vi "SFCS_GET_IMEI_IPEI_CMP_LBL.vi"() -> ()   [LabVIEW 2011]
uses:
  Instance           4 34Saved   SFCS_GET_IMEI_IPEI_CMP_LBL .vi
  Instance           8 34Saved   SFCS_GET_IMEI_IPEI_CMP_LBL .vi
  Instance           9 34Saved   SFCS_GET_IMEI_IPEI_CMP_LBL .vi
  Instance          10 34Saved   SFCS_GET_IMEI_IPEI_CMP_LBL .vi
  Instance          11 34Saved   SFCS_GET_IMEI_IPEI_CMP_LBL .vi
  Instance          14 34Saved   SFCS_GET_IMEI_IPEI_CMP_LBL .vi
panel:
  out "Found barcode label info?":bool
  out "IPEI_IMEI_Label":string
  out "SFCS_IPEI_IMEI":string
  out "SN":string
  out "SeqNo":i32
  out "Sequence":string
  out "Category":string
  out "STAGE":string
  out "SFCS_IP":string
  out "BEGIN TIME":u32
  # "KT300W/KT300M Get IPEI /IMEI from ShopFlow\n需網路連線至ShopFlow 取得IPEI /IMEI"
  # "2013-3-28"
  # "Step1: Get the IPEI or IMEI from a remote Server by issuing SN\n\nStep2: Auto Comapre with Label content and SN of Database"
  # "系統會自動比對Shoflow 的IPEI/IMEI 是否與條碼一致"
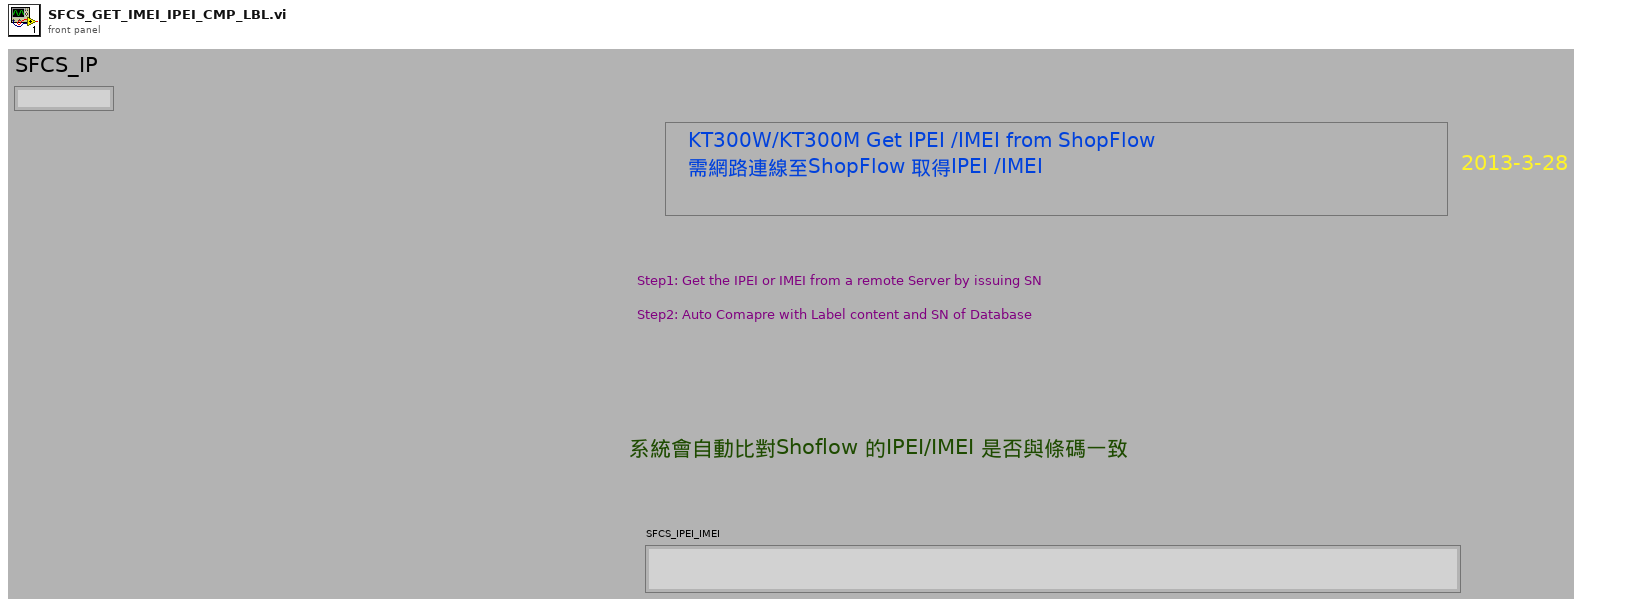
[diagram p1: front panel]
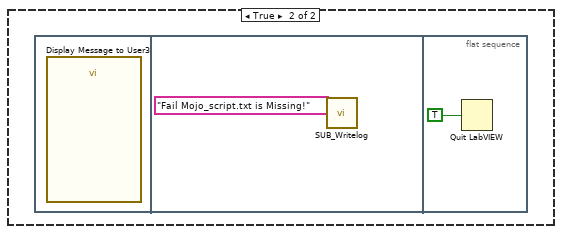
[diagram p5: hidden frame]
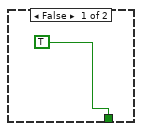
[diagram p8: hidden frame]
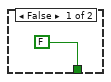
[diagram p9: hidden frame]
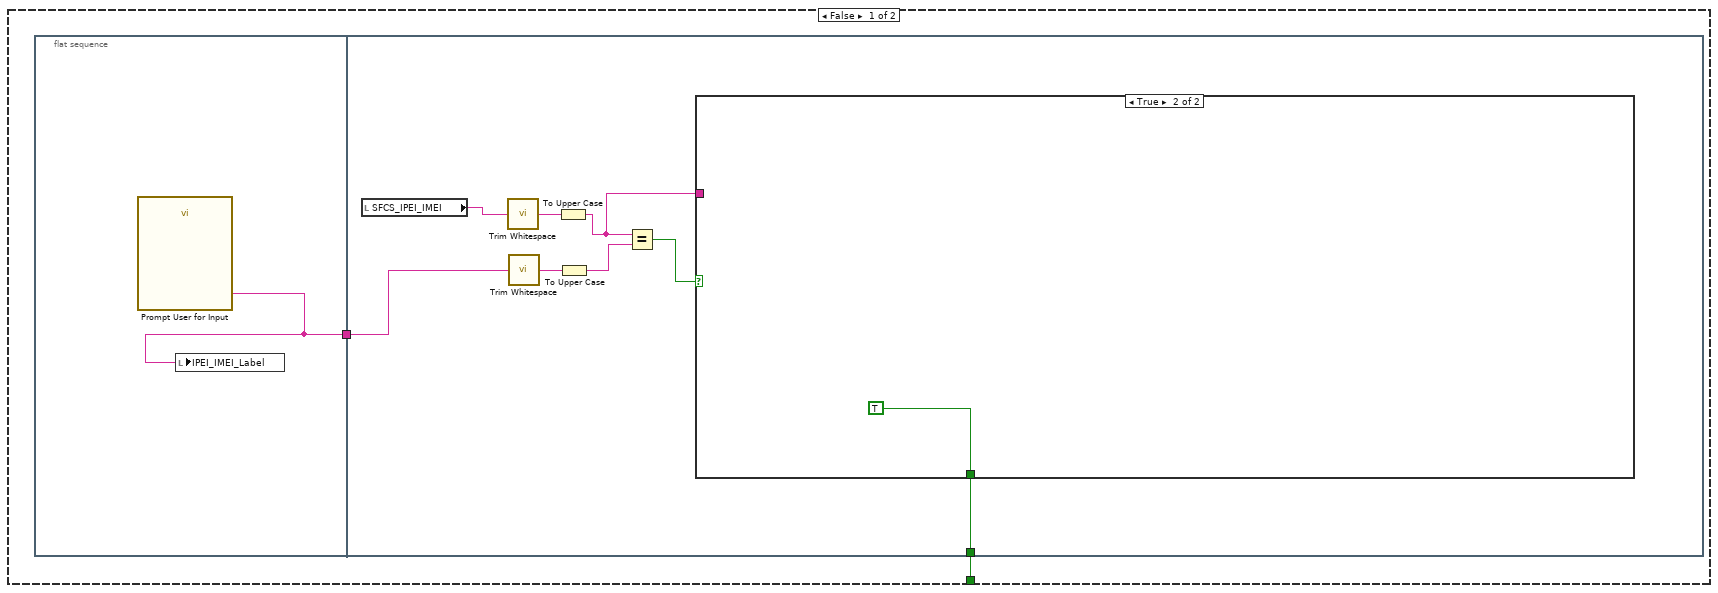
[diagram p10: hidden frame]
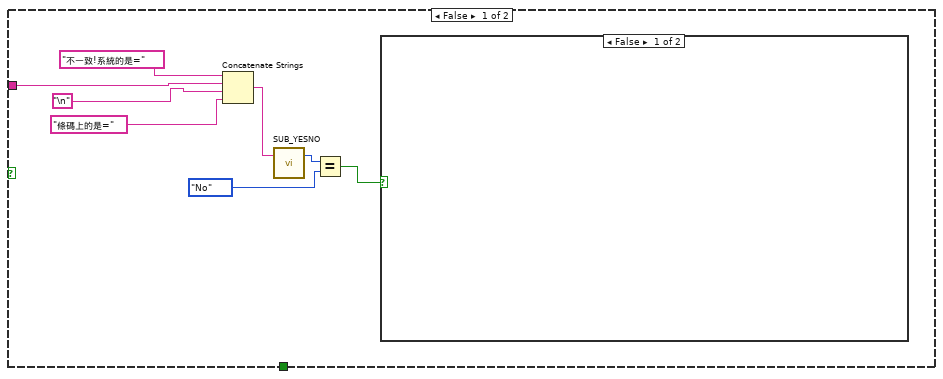
[diagram p11: hidden frame]
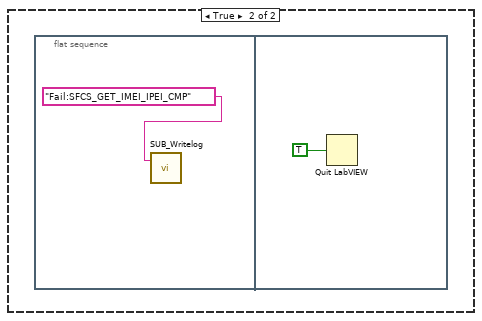
[diagram p12: hidden frame]
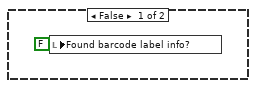
[diagram p13: hidden frame]
diagram:
  n1 = flat-sequence {
    tunnel: [w15] -> w1
    tunnel: w1 -> [w36]
    frame #0 {
      n2 = Tick Count (ms)() -> (millisecond timer value=→"BEGIN TIME":u32)
    }
    frame #1 {
      n3 = local write "Found barcode label info?"(FALSE ("Found barcode label info?")) -> ()
    }
    frame #2 {
      w4 = "barcode.LOG" ("Search Filename in Folder")
      n4 = call "SUB_SearchFile_inFolder.vi"("Search Filename in Folder"=w4) -> ("File Existing True/Flase"=w5:bool)  [unwired: 1 in]
      n5 = case shown="True" w5 {
        tunnel: w4 -> [_ w10]
        frame False {
        }
        frame True {
          n6 = call "SUB_Read_specifFile.vi"("name or relative path"=w10) -> ("text"=w9:string)  [unwired: 1 in, 1 out]
          n7 = call "SUB_FindSpecificString.vi"("Find this String"="IPEI_IMEI=", "String data"=w9) -> ("before \"; \" string"=→"IPEI_IMEI_Label":string, "Found"=→"Found barcode label info?":bool)  [unwired: 2 in]
        }
      }
    }
    frame #3 {
      n8 = call "SUB_SearchFile_inFolder.vi"("Search Filename in Folder"="SFCS_INFO.LOG") -> ("File Existing True/Flase"=w11:bool)  [unwired: 1 in]
      n9 = case shown="False" w11 {
        frame False {
          n10 = flat-sequence {
            frame #0 {
              n11 = call "Display Message to User"() -> ()  [unwired: 10 in, 2 out]
            }
            frame #1 {
              n12 = call "SUB_Writelog.vi"("Pass/Fail"="Fail :Please Do Check Route First !") -> ()  [unwired: 2 in]
            }
            frame #2 {
              n13 = Quit LabVIEW(quit? (T)=TRUE) -> ()
            }
          }
        }
        frame True {
        }
      }
    }
    frame #4 {
      n14 = call "SUB_ReadScript_File.vi"("Script FileName"="konftel_sfcs_misc.TXT") -> ("error out"=w19:errorcluster, "text"=w15:string)  [unwired: 1 in]
      n15 = Unbundle By Name(w19) -> ("code"=w18:i32)
      n16 = Not Equal To 0?(x=w18) -> (x != 0?=w17:bool)
      n17 = case shown="False" w17 {
        tunnel: w15 -> [w20 _]
        frame False {
          n18 = flat-sequence {
            tunnel: w20 -> [w26]
            frame #0 {
              n19 = To Upper Case(1:"SFCS_IP=" ("string")) -> (0:w30:string)
              n20 = To Upper Case(1:w26) -> (0:w31:string)
              n21 = call <vilib>:"Trim Whitespace.vi"("string"=w30) -> ("trimmed string"=w28:string)  [unwired: 1 in]
              n22 = call <vilib>:"Trim Whitespace.vi"("string"=w31) -> ("trimmed string"=w27:string)  [unwired: 1 in]
              n23 = Match Pattern(string=w27, regular expression=w28) -> (after substring=w25:string)  [unwired: 1 in, 3 out]
              n24 = Match Pattern(string=w25, regular expression=";") -> (before substring=w23:string)  [unwired: 1 in, 3 out]
              "SFCS_IP" <- w23
              n25 = Equal?(x=w23, y="") -> (x = y?=w21:bool)
              n26 = case shown="True" w21 {
                frame False {
                }
                frame True {
                  n27 = flat-sequence {
                    frame #0 {
                      n28 = call "Display Message to User2"() -> ()  [unwired: 10 in, 2 out]
                    }
                    frame #1 {
                      n29 = call "SUB_Writelog.vi"("Pass/Fail"="Fail Not Found SFCS_IP=\"xx.xx.xx.xx\" in Mojo_script.txt !") -> ()  [unwired: 2 in]
                    }
                    frame #2 {
                      n30 = Quit LabVIEW(quit? (T)=TRUE) -> ()
                    }
                  }
                }
              }
            }
          }
        }
        frame True {
          n31 = flat-sequence {
            frame #0 {
              n32 = call "Display Message to User3"() -> ()  [unwired: 10 in, 2 out]
            }
            frame #1 {
              n33 = call "SUB_Writelog.vi"("Pass/Fail"="Fail Mojo_script.txt is Missing!") -> ()  [unwired: 2 in]
            }
            frame #2 {
              n34 = Quit LabVIEW(quit? (T)=TRUE) -> ()
            }
          }
        }
      }
    }
    frame #5 {
      n35 = To Upper Case(1:"SFCS_STAGE=" ("string")) -> (0:w68:string)
      n36 = To Upper Case(1:w36) -> (0:w69:string)
      n37 = To Upper Case(1:"SFCS_IMEI_IPEI_Category=" ("string")) -> (0:w61:string)
      n38 = To Upper Case(1:w36) -> (0:w62:string)
      n39 = call <vilib>:"Trim Whitespace.vi"("string"=w68) -> ("trimmed string"=w67:string)  [unwired: 1 in]
      n40 = call <vilib>:"Trim Whitespace.vi"("string"=w69) -> ("trimmed string"=w66:string)  [unwired: 1 in]
      n41 = To Upper Case(1:"SFCS_Sequence=" ("string")) -> (0:w54:string)
      n42 = call <vilib>:"Trim Whitespace.vi"("string"=w61) -> ("trimmed string"=w60:string)  [unwired: 1 in]
      n43 = call <vilib>:"Trim Whitespace.vi"("string"=w62) -> ("trimmed string"=w59:string)  [unwired: 1 in]
      n44 = To Upper Case(1:w36) -> (0:w55:string)
      n45 = call <vilib>:"Trim Whitespace.vi"("string"=w54) -> ("trimmed string"=w53:string)  [unwired: 1 in]
      n46 = call <vilib>:"Trim Whitespace.vi"("string"=w55) -> ("trimmed string"=w52:string)  [unwired: 1 in]
      n47 = Match Pattern(string=w66, regular expression=w67) -> (after substring=w65:string)  [unwired: 1 in, 3 out]
      n48 = Match Pattern(string=w59, regular expression=w60) -> (after substring=w58:string)  [unwired: 1 in, 3 out]
      n49 = Match Pattern(string=w52, regular expression=w53) -> (after substring=w51:string)  [unwired: 1 in, 3 out]
      n50 = Match Pattern(string=w65, regular expression=";") -> (before substring=w48:string)  [unwired: 1 in, 3 out]
      "STAGE" <- w48
      n51 = Match Pattern(string=w58, regular expression=";") -> (before substring=w47:string)  [unwired: 1 in, 3 out]
      "Category" <- w47
      n52 = Match Pattern(string=w51, regular expression=";") -> (before substring=w38:string)  [unwired: 1 in, 3 out]
      "Sequence" <- w38
      n53 = Decimal String To Number(string=w38) -> (number=→"SeqNo":i32)  [unwired: 2 in, 1 out]
      n54 = Not Equal?(x=w47, y="") -> (x != y?=w42:bool)
      n55 = Not Equal?(x=w48, y="") -> (x != y?=w43:bool)
      n56 = Not Equal?(x=w38, y="") -> (x != y?=w40:bool)
      n57 = And(x=w43, y=w42) -> (x .and. y?=w41:bool)
      n58 = And(x=w41, y=w40) -> (x .and. y?=w39:bool)
      n59 = case shown="False" w39 {
        frame False {
          n60 = flat-sequence {
            frame #0 {
              n61 = call "Display Message to User4"() -> ()  [unwired: 10 in, 2 out]
            }
            frame #1 {
              n62 = call "SUB_Writelog.vi"("Pass/Fail"="Fail :Stage,Category,Sequence not define in script file!") -> ()  [unwired: 2 in]
            }
            frame #2 {
              n63 = Quit LabVIEW(quit? (T)=TRUE) -> ()
            }
          }
        }
        frame True {
        }
      }
    }
    frame #6 {
      n64 = call "SUB_Read_specifFile.vi"("name or relative path"="SFCS_INFO.LOG") -> ("error out"=w82:errorcluster, "text"=w81:string)  [unwired: 1 in]
      n65 = Unbundle By Name(w82) -> ("code"=w79:i32)
      n66 = call "SUB_FindSpecificString.vi"("Find this String"="USN=", "String data"=w81) -> ("before \"; \" string"=→"SN":string, "Found"=w77:bool)  [unwired: 2 in]
      n67 = Equal?(x=w79, y=0) -> (x = y?=w74:bool)
      n68 = Equal?(x=w77, y=TRUE) -> (x = y?=w75:bool)
      n69 = And(x=w75, y=w74) -> (x .and. y?=w72:bool)
      n70 = case shown="False" w72 {
        frame False {
          n71 = flat-sequence {
            frame #0 {
              n72 = call "Display Message to User5"() -> ()  [unwired: 10 in, 2 out]
            }
            frame #1 {
              n73 = call "SUB_Writelog.vi"("Pass/Fail"="Fail :Something is wrong in SFCS_INFO.LOG") -> ()  [unwired: 2 in]
            }
            frame #2 {
              n74 = Quit LabVIEW(quit? (T)=TRUE) -> ()
            }
          }
        }
        frame True {
        }
      }
    }
    frame #7 {
      n75 = while {
        stop <- w88 stop-if-true
        n76 = local read "Category"() -> (w91:string)
        n77 = local read "SeqNo"() -> (w90:i32)
        n78 = local read "SN"() -> (w93:string)
        n79 = local read "STAGE"() -> (w92:string)
        n80 = local read "SFCS_IP"() -> (w94:string)
        n81 = call "SUB_SFCS_GetUSNItem.vi"("URL"=w94, "SN"=w93, "Stage"=w92, "CATEGORY"=w91, "SEQ"=w90) -> ("Status"=w86:string)
        n82 = String Length(string=w86) -> (length=w102:i32)
        n83 = call "SUB_FindSpecificString.vi"("Find this String"="FAIL") -> ("Found"=w97:bool)  [unwired: 3 in, 1 out]
        n84 = call "SUB_FindSpecificString.vi"("Find this String"="NG", "String data"=w86) -> ("Found"=w99:bool)  [unwired: 2 in, 1 out]
        n85 = call <vilib>:"Trim Whitespace.vi"("string"=w86) -> ("trimmed string"=w96:string)  [unwired: 1 in]
        n86 = Less?(x=w102, y=3) -> (x < y?=w98:bool)
        n87 = To Upper Case(1:w96) -> (0:→"SFCS_IPEI_IMEI":string)
        n88 = Or(x=w99, y=w98) -> (x .or. y?=w89:bool)
        n89 = Or(x=w89, y=w97) -> (x .or. y?=w87:bool)
        n90 = case shown="True" w87 {
          tunnel: [TRUE w106] -> w88
          tunnel: w86 -> [_ w105]
          frame False {
          }
          frame True {
            n91 = call "SUB_YESNO.vi"("Debug View"=w105, "Status"="ShopFlow 要不到資料,網址需正確.網路需連線.") -> ("yes/no"=w109:enum32{"No Selection", "Yes", "No", "None"})  [unwired: 1 in]
            n92 = Equal?(x=w109, y=enum32{"No Selection", "Yes", "No", "None"}."No") -> (x = y?=w107:bool)
            n93 = case shown="True" w107 {
              tunnel: [FALSE w112] -> w106
              frame False {
              }
              frame True {
                n94 = flat-sequence {
                  tunnel: [w114] -> w112
                  frame #0 {
                    n95 = call "SUB_Writelog.vi"("Pass/Fail"="FailSFCS_GET_IMEI_IPEI_CMP_LBL") -> ()  [unwired: 2 in]
                  }
                  frame #1 {
                    w114 = TRUE ("quit? (T)")
                    n96 = Quit LabVIEW(quit? (T)=w114) -> ()
                  }
                }
              }
            }
          }
        }
      }
    }
    frame #8 {
      n97 = while {
        stop <- w115 stop-if-true
        n98 = local read "Found barcode label info?"() -> (w116:bool)
        n99 = case shown="True" w116 {
          tunnel: [w117 _] -> w115
          frame False {
            n100 = flat-sequence {
              tunnel: [w119] -> w118
              tunnel: w118 -> [w124]
              tunnel: [w121] -> w117
              frame #0 {
                n101 = call "Prompt User for Input"() -> ("IEPI_IMEI"=w119:string)  [unwired: 17 in, 2 out]
                n102 = local write "IPEI_IMEI_Label"(w119) -> ()
              }
              frame #1 {
                n103 = local read "SFCS_IPEI_IMEI"() -> (w126:string)
                n104 = call <vilib>:"Trim Whitespace.vi"("string"=w126) -> ("trimmed string"=w127:string)  [unwired: 1 in]
                n105 = call <vilib>:"Trim Whitespace.vi"("string"=w124) -> ("trimmed string"=w125:string)  [unwired: 1 in]
                n106 = To Upper Case(1:w127) -> (0:w120:string)
                n107 = To Upper Case(1:w125) -> (0:w123:string)
                n108 = Equal?(x=w120, y=w123) -> (x = y?=w122:bool)
                n109 = case shown="True" w122 {
                  tunnel: [_ TRUE] -> w121
                  tunnel: w120 -> [w134 _]
                  frame False {
                    n110 = Concatenate Strings("不一致!系統的是=", w134, "\n", "條碼上的是=") -> (w131:string)
                    n111 = call "SUB_YESNO.vi"("Status"=w131) -> ("yes/no"=w130:enum32{"No Selection", "Yes", "No", "None"})  [unwired: 2 in]
                    n112 = Equal?(x=w130, y=enum32{"No Selection", "Yes", "No", "None"}."No") -> (x = y?=w128:bool)
                    n113 = case shown="False" w128 {
                      frame False {
                      }
                      frame True {
                        n114 = flat-sequence {
                          frame #0 {
                            n115 = call "SUB_Writelog.vi"("Pass/Fail"="Fail:SFCS_GET_IMEI_IPEI_CMP") -> ()  [unwired: 2 in]
                          }
                          frame #1 {
                            n116 = Quit LabVIEW(quit? (T)=TRUE) -> ()
                          }
                        }
                      }
                    }
                  }
                  frame True {
                  }
                }
              }
            }
          }
          frame True {
            n117 = local read "IPEI_IMEI_Label"() -> (w143:string)
            n118 = local read "SFCS_IPEI_IMEI"() -> (w139:string)
            n119 = call <vilib>:"Trim Whitespace.vi"("string"=w143) -> ("trimmed string"=w144:string)  [unwired: 1 in]
            n120 = call <vilib>:"Trim Whitespace.vi"("string"=w139) -> ("trimmed string"=w145:string)  [unwired: 1 in]
            n121 = To Upper Case(1:w144) -> (0:w141:string)
            n122 = To Upper Case(1:w145) -> (0:w142:string)
            n123 = Equal?(x=w142, y=w141) -> (x = y?=w140:bool)
            n124 = case shown="True" w140 {
              tunnel: w139 -> [_ w147]
              frame False {
                n125 = local write "Found barcode label info?"(FALSE ("Found barcode label info?")) -> ()
              }
              frame True {
                n126 = flat-sequence {
                  tunnel: w147 -> [w157]
                  frame #0 {
                    n127 = local read "BEGIN TIME"() -> (w155:u32)
                    n128 = Tick Count (ms)() -> (millisecond timer value=w154:u32)
                    n129 = call "SUB_CAL_TESTTIME.vi"("Test Item name"="SFCS_GET_IMEI_IPEI_CMP_LBL", "Stop tick time"=w154, "Start tick time"=w155) -> ("Test Time output"=w152:string)  [unwired: 2 in]
                    n130 = Concatenate Strings("IPEI_IMEI=" ("string"), w157, ";", w152) -> (w150:string)
                    n131 = Concatenate Strings("Pass:SFCS_GET_IMEI_IPEI_CMP_LBL", "\n", w150) -> (w151:string)
                    n132 = call "SUB_Writelog.vi"("Pass/Fail"=w151) -> ()  [unwired: 2 in]
                  }
                  frame #1 {
                    n133 = Quit LabVIEW(quit? (T)=TRUE) -> ()
                  }
                }
              }
            }
          }
        }
      }
    }
    frame #9 {
      n134 = local read "SFCS_IPEI_IMEI"() -> (w161:string)
      n135 = local read "BEGIN TIME"() -> (w160:u32)
      n136 = Tick Count (ms)() -> (millisecond timer value=w168:u32)
      n137 = call "SUB_CAL_TESTTIME.vi"("Test Item name"="SFCS_GET_IMEI_IPEI_CMP_LBL", "Stop tick time"=w168, "Start tick time"=w160) -> ("Test Time output"=w166:string)  [unwired: 2 in]
      n138 = Concatenate Strings("IPEI_IMEI=" ("string"), w161, ";", w166) -> (w164:string)
      n139 = Concatenate Strings("PassSFCS_GET_IMEI_IPEI_CMP_LBL", "\n", w164) -> (w165:string)
      n140 = call "SUB_Writelog.vi"("Pass/Fail"=w165) -> ()  [unwired: 2 in]
    }
    frame #10 {
      n141 = Quit LabVIEW(quit? (T)=TRUE) -> ()
    }
  }
